vi "FlatToRichcif_manager_ClockConversionArray.vi"(5 "OutputClusterType":T1, 11 "InputCluster":T4) -> (3 "OutputCluster":T1)   [LabVIEW 2021, in "CIF_Manager_client.lvlib"]
uses:
  CIF_Manager_client.lvlib
  cif_manager_ClockConversionArray_Flat.ctl
  cif_manager_ClockConversion_Flat.ctl
  cif_manager_TimePair_Flat.ctl
  cif_manager_ClockConversionArray.ctl
  cif_manager_ClockConversion.ctl
  cif_manager_TimePair.ctl
  FlatToRichcif_manager_TimePair.vi
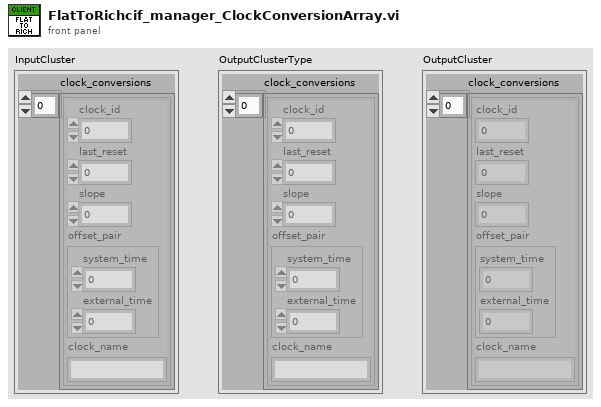
[diagram p1: front panel]
types:
  T1 = typedef "CIF_Manager_client.lvlib/cif_manager_ClockConversionArray.ctl" = cluster{"clock_conversions":T2[]}
  T2 = typedef "CIF_Manager_client.lvlib/cif_manager_ClockConversion.ctl" = cluster{"clock_id":u32, "last_reset":i64, "slope":dbl, "offset_pair":T3, "clock_name":string}
  T3 = typedef "CIF_Manager_client.lvlib/cif_manager_TimePair.ctl" = cluster{"system_time":i64, "external_time":i64}
  T4 = typedef "CIF_Manager_client.lvlib/cif_manager_ClockConversionArray_Flat.ctl" = cluster{"clock_conversions":T5[]}
  T5 = typedef "CIF_Manager_client.lvlib/cif_manager_ClockConversion_Flat.ctl" = cluster{"clock_id":u32, "last_reset":i64, "slope":dbl, "offset_pair":T6, "clock_name":string}
  T6 = typedef "CIF_Manager_client.lvlib/cif_manager_TimePair_Flat.ctl" = cluster{"system_time":i64, "external_time":i64}
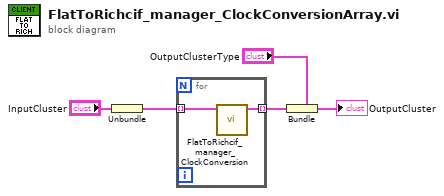
[diagram p0: block diagram]
diagram:
  n1 = Unbundle "Unbundle"("InputCluster") -> ("clock_conversions"=w2:T5[])
  n2 = for {
    tunnel: w2 -> [w7] mode=indexing
    tunnel: [w6] -> w1 mode=indexing
    n3 = call "FlatToRichcif_manager_ClockConversion.vi"("InputCluster"=w7) -> ("OutputCluster"=w6:T2)  [unwired: 10 in]
  }
  n4 = Bundle "Bundle"(cluster="OutputClusterType", "clock_conversions"=w1) -> (→"OutputCluster":T1)
